vi "Act.vi"(4 "V":i8, 5 "InWorld":i8[][](array[numeric])=[[0, 0, 0, 0, 0, 0, 0, 0, 0, 0], [0, 0, 0, 0, 0, 0, 0, 0, 0, 0], [0, 0, 0, 0, 0, 0, 0, 0, 0, 0], [0, 1, 1, 1, 1, 1, 1, 1, 1, 0], [0, 1, 1, 1, 1, 1, 1, 1, 1, 0], [0, 1, 1, 1, 1, 1, 1, 1, 1, 0], [0, 1, 1, 1, 1, 1, 1, 1, 1, 0], [0, 1, 1, 1, 1, 1, 1, 1, 1, 0], [0, 0, 0, 0, 0, 0, 0, 0, 0, 0], [0, 0, 0, 0, 0, 0, 0, 0, 0, 0]], 6 "E_in":i8, 7 "Y_in":i8, 8 "X_in":i8) -> (0 "Outworld":i8[][](array[numeric]), 1 "E_out":i8, 2 "Y_out":i8, 3 "X_out":i8)   [LabVIEW 2014]
doc: "This VI moves the robot based on the following code:\n6 7 8\n5 0 1\n4 3 2"
panel:
  # "V Code\n  6 7 8\n  5 0 1\n  4 3 2"
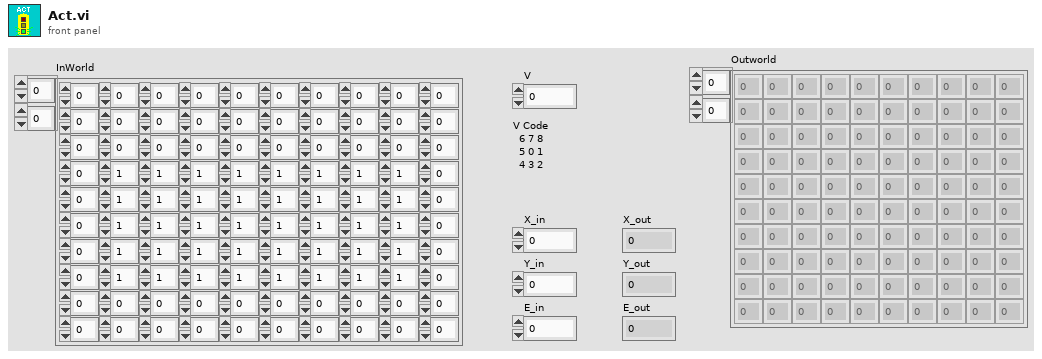
[diagram p1: front panel]
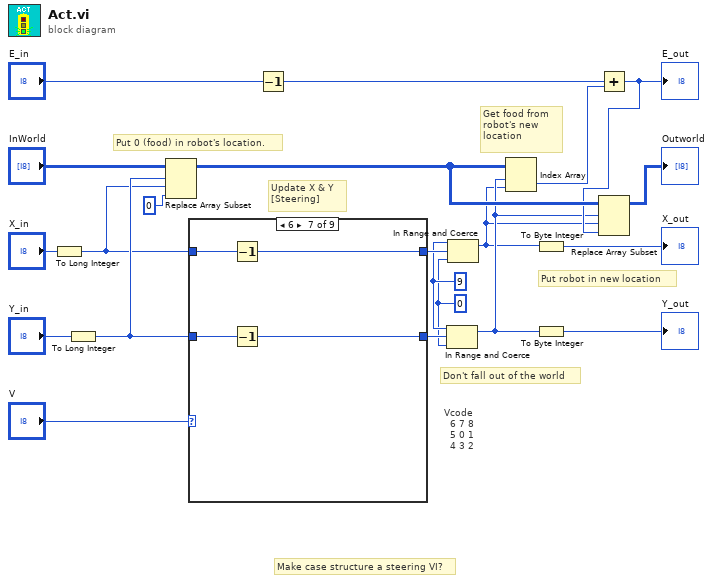
[diagram p0: block diagram]
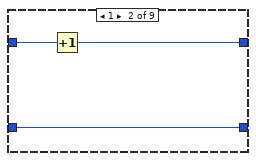
[diagram p3: hidden frame]
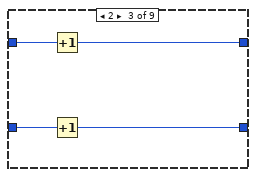
[diagram p4: hidden frame]
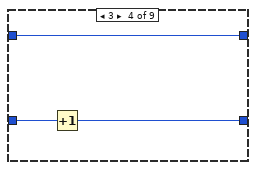
[diagram p5: hidden frame]
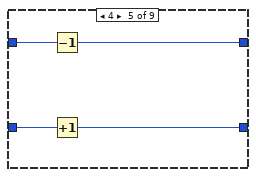
[diagram p6: hidden frame]
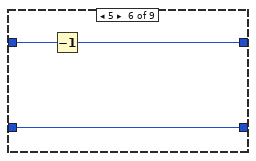
[diagram p7: hidden frame]
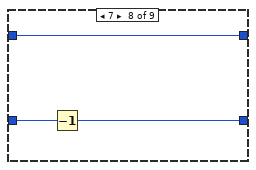
[diagram p8: hidden frame]
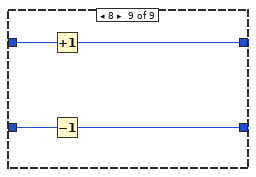
[diagram p9: hidden frame]
diagram:
  w17 = 0
  w18 = 9
  # "Don't fall out of the world"
  # "Put robot in new location"
  # "Get food from \nrobot's new \nlocation"
  # "Update X & Y \n[Steering]"
  # "Put 0 (food) in robot's location."
  # "Make case structure a steering VI?"
  # "Vcode\n  6 7 8\n  5 0 1\n  4 3 2"
  n1 = To Long Integer(number="X_in") -> (32bit integer=w3:i32)
  n2 = To Long Integer(number="Y_in") -> (32bit integer=w4:i32)
  n3 = Replace Array Subset(array="InWorld", new element=i8 0 ("new element/subarray"), index (row)=w4, index (col)=w3) -> (w10:i8[][])
  n4 = case shown="6" "V" {
    tunnel: w3 -> [w22 w26 w30 w31 w34 w40 w44 w45 w51]
    tunnel: w4 -> [w23 w24 w28 w33 w37 w38 w42 w47 w49]
    tunnel: [w22 w25 w29 w31 w35 w39 w43 w45 w50] -> w20
    tunnel: [w23 w24 w27 w32 w36 w38 w41 w46 w48] -> w19
    frame 0, Default {
    }
    frame 1 {
      n5 = Increment(x=w26) -> (x+1=w25:i32)
    }
    frame 2 {
      n6 = Increment(x=w30) -> (x+1=w29:i32)
      n7 = Increment(x=w28) -> (x+1=w27:i32)
    }
    frame 3 {
      n8 = Increment(x=w33) -> (x+1=w32:i32)
    }
    frame 4 {
      n9 = Decrement(x=w34) -> (x-1=w35:i32)
      n10 = Increment(x=w37) -> (x+1=w36:i32)
    }
    frame 5 {
      n11 = Decrement(x=w40) -> (x-1=w39:i32)
    }
    frame 6 {
      n12 = Decrement(x=w44) -> (x-1=w43:i32)
      n13 = Decrement(x=w42) -> (x-1=w41:i32)
    }
    frame 7 {
      n14 = Decrement(x=w47) -> (x-1=w46:i32)
    }
    frame 8 {
      n15 = Increment(x=w51) -> (x+1=w50:i32)
      n16 = Decrement(x=w49) -> (x-1=w48:i32)
    }
  }
  n17 = Decrement(x="E_in") -> (x-1=w15:i8)
  n18 = In Range and Coerce(upper limit=w18, x=w19, lower limit=w17) -> (coerced(x)=w2:i32)  [unwired: 1 out]
  n19 = In Range and Coerce(upper limit=w18, x=w20, lower limit=w17) -> (coerced(x)=w1:i32)  [unwired: 1 out]
  n20 = Index Array(array=w10, index (row)=w2, index (col)=w1) -> (element=w12:i8)
  n21 = To Byte Integer(number=w1) -> (8bit integer=→"X_out":i8)
  n22 = To Byte Integer(number=w2) -> (8bit integer=→"Y_out":i8)
  n23 = Add(x=w15, y=w12) -> (x+y=w9:i8)
  "E_out" <- w9
  n24 = Replace Array Subset(array=w10, new element=w9, index (row)=w2, index (col)=w1) -> (→"Outworld":i8[][])
